vi "TestExecuteValueChangeSubscription_RejectRepeats.vi"(8 "error in (no error)":errorcluster, 11 "TestCase in":refnum<class "TestSubscriptionPolicy.lvclass">) -> (0 "error out":errorcluster, 3 "TestCase out":refnum<class "TestSubscriptionPolicy.lvclass">)   [LabVIEW 2017, in "TestSubscriptionPolicy.lvclass"]
uses:
  TestSubscriptionPolicy.lvclass
  ValueChangeSubscription/ValueChangeSubscription.lvclass/ValueChangeSubscription.ctl
  Transport/QueueTransport/QueueTransport.lvclass/QueueTransport.ctl
  IMediator/ISubscriptionPolicy/ISubscriptionPolicy.lvclass/ISubscriptionPolicy.ctl
  Transport/QueueTransport/QueueTransport.lvclass
  C:/Git/mva-framework/Framework/IMediator/ITransport/ITransport.lvclass
  ValueChangeSubscription/ValueChangeSubscription.lvclass
  C:/Git/mva-framework/Framework/IMediator/ISubscriptionPolicy/ISubscriptionPolicy.lvclass
  <vilib>/Utility/error.llb/Error Cluster From Error Code.vi
  IMediator/ISubscriptionPolicy/ISubscriptionPolicy.lvclass
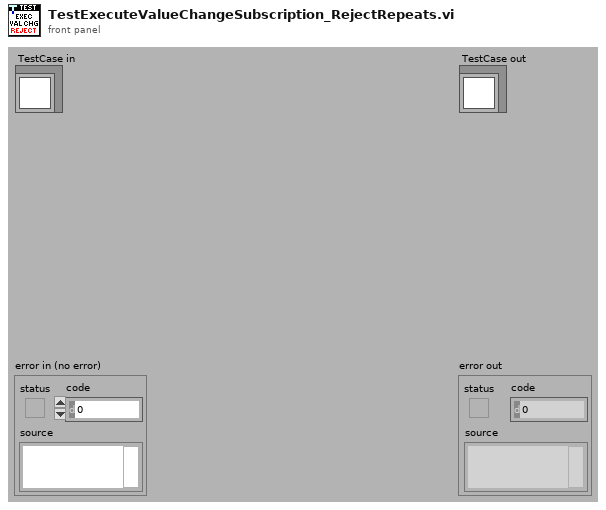
[diagram p1: front panel]
types:
  T1 = typedef "IMediator.lvlib/ISubscriptionPolicy.lvclass/ISubscriptionPolicy Reference.ctl" = refnum<data-value>
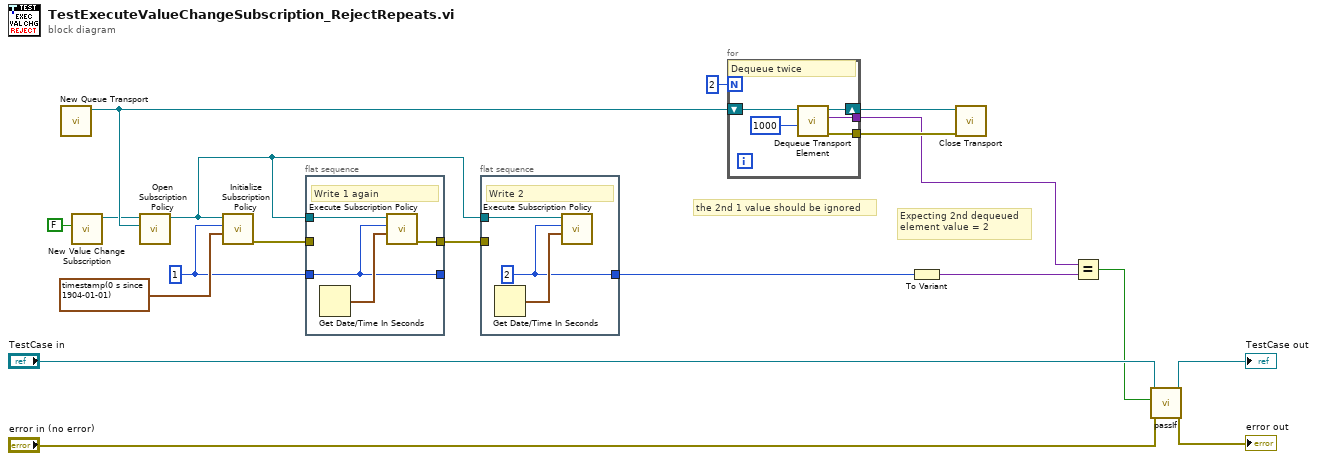
[diagram p0: block diagram]
diagram:
  w8 = 1
  # "the 2nd 1 value should be ignored"
  # "Expecting 2nd dequeued\nelement value = 2"
  n1 = call "New Queue Transport.vi"() -> ("QueueTransport"=w15:refnum<class "QueueTransport.lvclass">)  [unwired: 10 in, 1 out]
  n2 = call "New Value Change Subscription.vi"("Ignore Past Updates? (F)"=FALSE) -> ("ValueChangeSubscription Out"=w12:refnum<class "ValueChangeSubscription.lvclass">)  [unwired: 10 in]
  n3 = call "Open Subscription Policy.vi"("Transport"=w15, "SubscriptionPolicy"=w12) -> ("Subscription Policy"=w5:T1)  [unwired: 8 in, 1 out]
  n4 = call "Initialize Subscription Policy.vi"("Last Publish Time"=timestamp(0 s since 1904-01-01), "Last Topic Value"=w8, "Subscription Policy"=w5) -> ("Error Out (Do Not Subscribe?)"=w6:errorcluster)  [unwired: 8 in]
  n5 = flat-sequence {
    tunnel: w8 -> [w21]
    tunnel: w5 -> [w22]
    tunnel: w6 -> [_]
    tunnel: [w21] -> _
    tunnel: [w20] -> w2
    frame #0 {
      # "Write 1 again"
      n6 = Get Date/Time In Seconds() -> (seconds since 1Jan1904=w23:timestamp)
      n7 = call "Execute Subscription Policy.vi"("Publish Time"=w23, "New Topic Value"=w21, "Subscription Policy"=w22) -> ("error out (Unsubscribe?)"=w20:errorcluster)  [unwired: 8 in]
    }
  }
  n8 = flat-sequence {
    tunnel: w5 -> [w25]
    tunnel: [w24] -> w4
    tunnel: w2 -> [_]
    frame #0 {
      w24 = 2
      # "Write 2"
      n9 = Get Date/Time In Seconds() -> (seconds since 1Jan1904=w26:timestamp)
      n10 = call "Execute Subscription Policy.vi"("Publish Time"=w26, "New Topic Value"=w24, "Subscription Policy"=w25) -> ()  [unwired: 8 in, 1 out]
    }
  }
  n11 = for {
    N: 2 -> [_]
    tunnel: [w29] -> w1
    tunnel: [w27] -> w13
    shift-right: [w28] -> w14
    shift-left: w15 -> [w31]
    # "Dequeue twice"
    n12 = call "Dequeue Transport Element.vi"("Timeout In ms (-1)"=1000, "QueueTransport in"=w31) -> ("error out"=w27:errorcluster, "Data"=w29:variant, "QueueTransport out"=w28:refnum<class "QueueTransport.lvclass">)  [unwired: 6 in, 1 out]
  }
  n13 = To Variant(anything=w4) -> (Variant=w10:variant)
  n14 = call-dynamic "Close Transport.vi"("error in (no error)"=w13, "QueueTransport in"=w14) -> ()  [unwired: 9 in, 1 out]
  n15 = Equal?(x=w1, y=w10) -> (x = y?=w7:bool)
  n16 = call-dynamic "passIf.vi"("error in (no error)"="error in (no error)", "pass"=w7, "TestCase in"="TestCase in") -> ("error out"=→"error out":errorcluster, "TestCase out"=→"TestCase out":refnum<class "TestSubscriptionPolicy.lvclass">)  [unwired: 7 in]
